vi "MotorQuery.vi"(3 "VISA in":refnum<visa-resource-name>, 7 "Command":T1(ring), 9 "entrée d'erreur":errorcluster) -> (0 "VISA out":refnum<visa-resource-name>, 1 "Error Code":i32, 2 "I32 Result":i32, 5 "TF Result":bool, 6 "sortie d'erreur":errorcluster)   [LabVIEW 2009]
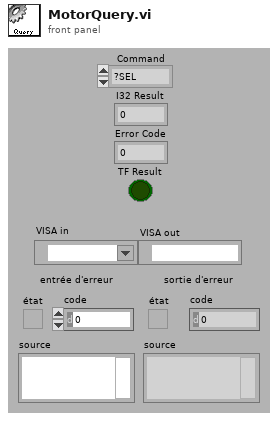
[diagram p1: front panel]
types:
  T1 = enum16{"?SEL", "?POS", "?VMIN", "?VMAX", "?ACC", "?MPAS", "?INT", "?JEU", "?OFFSET", "?L", "?FDC", "??", "?ST", "?MVT"}
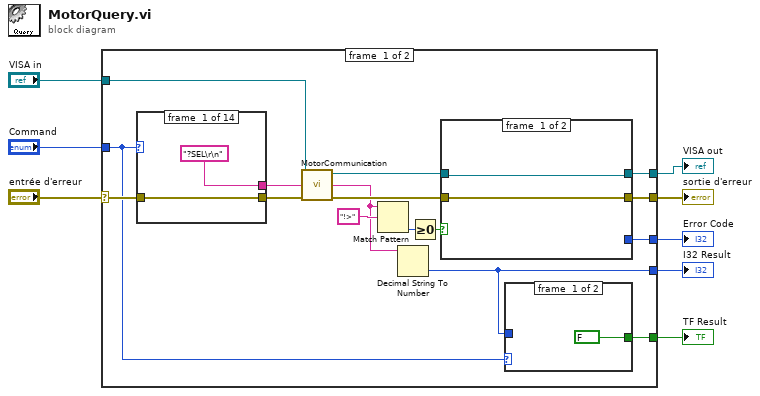
[diagram p0: block diagram]
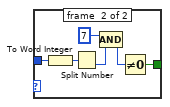
[diagram p2: hidden frame]
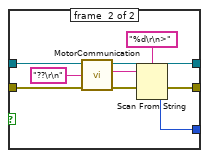
[diagram p3: hidden frame]
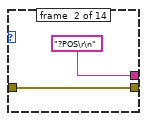
[diagram p4: hidden frame]
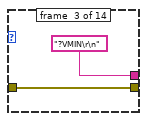
[diagram p5: hidden frame]
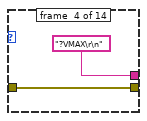
[diagram p6: hidden frame]
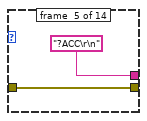
[diagram p7: hidden frame]
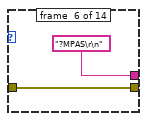
[diagram p8: hidden frame]
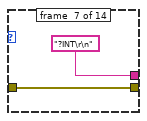
[diagram p9: hidden frame]
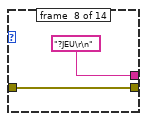
[diagram p10: hidden frame]
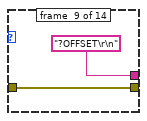
[diagram p11: hidden frame]
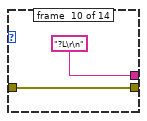
[diagram p12: hidden frame]
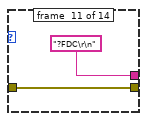
[diagram p13: hidden frame]
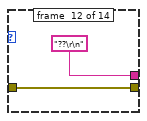
[diagram p14: hidden frame]
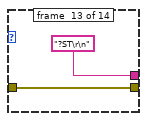
[diagram p15: hidden frame]
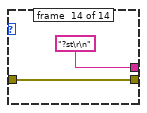
[diagram p16: hidden frame]
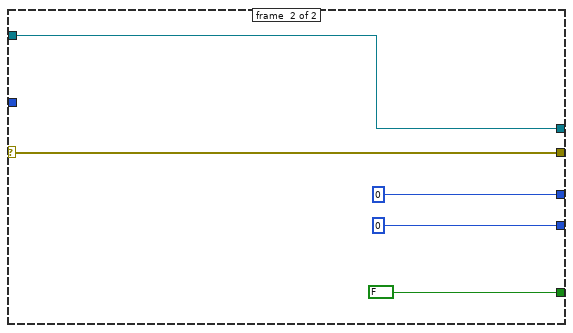
[diagram p17: hidden frame]
diagram:
  n1 = case shown="No Error" "entrée d'erreur" {
    selector: "entrée d'erreur" -> [w23 w76]
    tunnel: "Command" -> [w11 _]
    tunnel: "VISA in" -> [w15 w74]
    tunnel: [w17 0] -> w5
    tunnel: [w22 w74] -> w4
    tunnel: [w9 w76] -> w3
    tunnel: [w18 0] -> w2
    tunnel: [w19 FALSE] -> w1
    frame #0 {
      n2 = case shown="\"?MVT\"" w11 {
        tunnel: w23 -> [w44 w46 w48 w50 w52 w54 w56 w58 w60 w62 w64 w66 w68 w71]
        tunnel: ["?SEL\r\n" "?POS\r\n" "?VMIN\r\n" "?VMAX\r\n" "?ACC\r\n" "?MPAS\r\n" "?INT\r\n" "?JEU\r\n" "?OFFSET\r\n" "?L\r\n" "?FDC\r\n" "??\r\n" "?ST\r\n" "?st\r\n"] -> w14
        tunnel: [w44 w46 w48 w50 w52 w54 w56 w58 w60 w62 w64 w66 w68 w71] -> w10
        frame #0 {
        }
        frame #1 {
        }
        frame #2 {
        }
        frame #3 {
        }
        frame #4 {
        }
        frame #5 {
        }
        frame #6 {
        }
        frame #7 {
        }
        frame #8 {
        }
        frame #9 {
        }
        frame #10 {
        }
        frame #11 {
        }
        frame #12 {
        }
        frame #13 {
        }
      }
      n3 = call "MotorCommunication.vi"("Question"=w14, "error out"=w10, "COM Port in"=w15) -> ("error IO"=w16:errorcluster, "COM Port out"=w13:refnum<visa-resource-name>, "Answer"=w12:string)  [unwired: 4 out]
      n4 = Match Pattern(string=w12, regular expression="!>") -> (offset past match=w24:i32)  [unwired: 4 out]
      n5 = Decimal String To Number(string=w12) -> (number=w17:i32)  [unwired: 3 out]
      n6 = Greater Or Equal To 0?(x=w24) -> (x >= 0?=w20:bool)
      n7 = case "Structure Condition" shown="False" w20 {
        tunnel: w16 -> [w33 w40]
        tunnel: w13 -> [w34 w39]
        tunnel: [w33 w42] -> w9
        tunnel: [w34 w36] -> w22
        tunnel: [0 w41] -> w18
        frame #0 {
        }
        frame #1 {
          n8 = call "MotorCommunication.vi"("Question"="??\r\n" ("buffer à écrire"), "error out"=w40, "COM Port in"=w39) -> ("error IO"=w35:errorcluster, "COM Port out"=w36:refnum<visa-resource-name>, "Answer"=w37:string)  [unwired: 4 out]
          n9 = Scan From String(format string="%d\r\n>" ("chaîne de format"), input string=w37, error in=w35) -> (error out=w42:errorcluster, output 1=w41:i32)  [unwired: 1 in, 3 out]
        }
      }
      n10 = case shown="\"?MVT\"" w11 {
        tunnel: [FALSE w27] -> w19
        tunnel: w17 -> [_ w26]
        frame #0 {
        }
        frame #1 {
          n11 = To Word Integer(number=w26) -> (16bit integer=w31:i16)
          n12 = Split Number(x=w31) -> (lo(x)=w29:u8)  [unwired: 1 out]
          n13 = Compound Arithmetic op=AND(u8 7 ("valeur"), w29) -> (w30:u8)
          n14 = Not Equal To 0?(x=w30) -> (x != 0?=w27:bool)
        }
      }
    }
    frame #1 {
    }
  }
  "sortie d'erreur" <- w3
  "I32 Result" <- w5
  "VISA out" <- w4
  "Error Code" <- w2
  "TF Result" <- w1
